vi "AdaptToInputs.vi"(3 "Term Types":T1[](array[typedef]), 4 "XRef":refnum<vi>, 5 "State In":T4={"Enum Type"=variant(dbl 0.0), "Types Type"=variant(string ""), "Enum Names"=[], "Type Names"=[], "Typedef Name"="", "Typedef Path"=path ""}) -> (0 "Reply":string[](array[string]), 2 "State Out":T4={"Enum Type"=variant(dbl 0.0), "Types Type"=variant(string ""), "Enum Names"=[], "Type Names"=[], "Typedef Name"="", "Typedef Path"=path ""})   [LabVIEW 2015, in "Define-Tagged-Union.xnode"]
doc: "This ability VI is called by LabVIEW during type propagation so that your XNode may adapt itself to new input types. Term Types is an array of pairs of current Term IDs and the type descriptors corresponding to them. The type descriptors are taken from the signal connected to the terminal. Unwired terminals are not included in the array. Use Reply to inform LabVIEW of any actions it needs to take.\n\nDefault behavior: None.\n\nThis ability does not provide UI and OS messages are not handled."
uses:
  Define-Tagged-Union.xnode
  State.ctl
  <vilib>/XNodeSupport/XNodeTermTypeIDPair.ctl
  <vilib>/XNodeSupport/XNodeType.ctl
  <vilib>/XNodeSupport/XNodeString.ctl
  <vilib>/Erdos Miller/LV-Scripting/LV-Scripting.lvlib
  <vilib>/Utility/Data Type/NI_Data Type.lvlib
  <vilib>/XNodeSupport/NI_XNodeSupport.lvlib
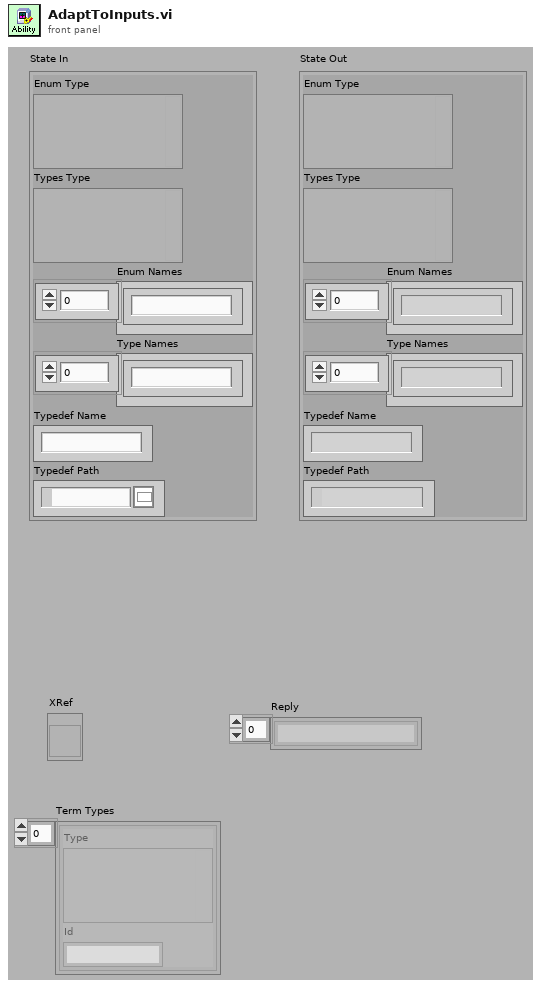
[diagram p1: front panel]
types:
  T1 = typedef "NI_XNodeSupport.lvlib/XNodeTermTypeIDPair.ctl" = cluster{"Type":T2, "Id":T3}
  T2 = typedef "NI_XNodeSupport.lvlib/XNodeType.ctl" = variant
  T3 = typedef "NI_XNodeSupport.lvlib/XNodeString.ctl" = string
  T4 = typedef "Define-Tagged-Union.xnode/State.ctl" = cluster{"Enum Type":variant, "Types Type":variant, "Enum Names":string[], "Type Names":string[], "Typedef Name":string, "Typedef Path":path}
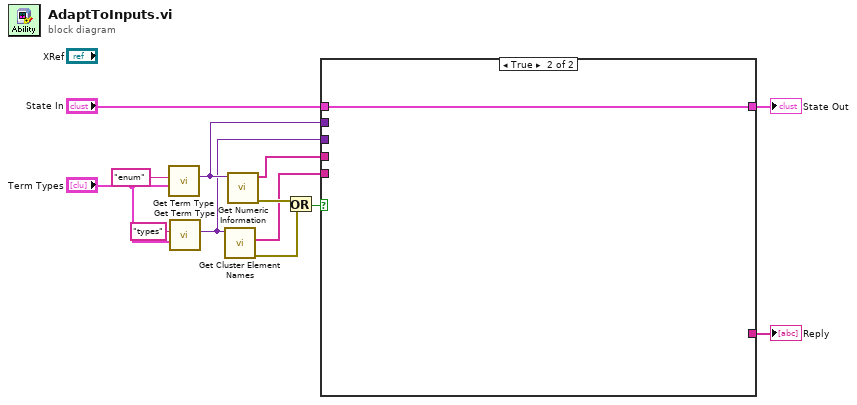
[diagram p0: block diagram]
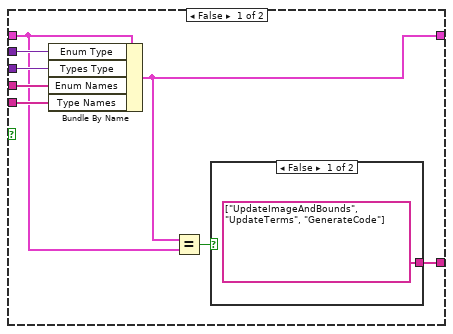
[diagram p2: hidden frame]
diagram:
  n1 = call <vilib>:"Get Term Type.vi"("Term Types"="Term Types", "ID"="enum") -> ("Type"=w4:variant)  [unwired: 9 in]
  n2 = call <vilib>:"Get Term Type.vi"("Term Types"="Term Types", "ID"="types") -> ("Type"=w3:variant)  [unwired: 9 in]
  n3 = call <vilib>:"Get Cluster Element Names.vi"("Cluster in"=w3) -> ("error out"=w2:errorcluster, "Names"=w1:string[])  [unwired: 8 in, 1 out]
  n4 = call <vilib>:"Get Numeric Information.vi"("Variant"=w4) -> ("error out"=w7:errorcluster, "Enum Names"=w5:string[])  [unwired: 7 in, 2 out]
  n5 = Or(x=w7, y=w2) -> (x .or. y?=w6:bool)
  n6 = case shown="True" w6 {
    tunnel: [w21 _] -> w11
    tunnel: "State In" -> [w15 w23]
    tunnel: [w16 w23] -> w10
    tunnel: w5 -> [w20 _]
    tunnel: w4 -> [w17 _]
    tunnel: w3 -> [w19 _]
    tunnel: w1 -> [w18 _]
    frame False {
      n7 = Bundle By Name(cluster=w15, "Enum Type"=w17, "Types Type"=w19, "Enum Names"=w20, "Type Names"=w18) -> (w16:T4)
      n8 = Equal?(x=w16, y=w15) -> (x = y?=w14:bool)
      n9 = case shown="False" w14 {
        tunnel: [string[] ["UpdateImageAndBounds", "UpdateTerms", "GenerateCode"] ("Reply") _] -> w21
        frame False {
        }
        frame True {
        }
      }
    }
    frame True {
    }
  }
  "Reply" <- w11
  "State Out" <- w10
